vi "Build Values Tree.vi"(7 "Tree":refnum<vi>, 11 "Types":T1[](array[typedef])) -> ()   [LabVIEW 2020, in "FlexBlocks.lvlib"]
uses:
  FlexBlocks.lvlib
  Type Descriptor.ctl
  Terminal Direction.ctl
  Value Mode.ctl
  Special Terminal.ctl
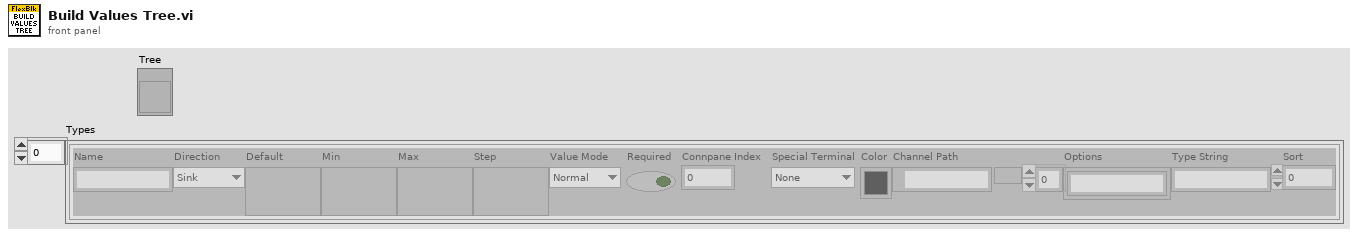
[diagram p1: front panel]
types:
  T1 = typedef "FlexBlocks.lvlib/Type Descriptor.ctl" = cluster{"Name":string, "Direction":T2, "Default":variant, "Min":variant, "Max":variant, "Step":variant, "Value Mode":T3, "Required":bool, "Connpane Index":i32, "Special Terminal":T4, "Color":u32, "Channel Path":path, "Options":string[], "Type String":string, "Sort":i32}
  T2 = typedef "FlexBlocks.lvlib/Terminal Direction.ctl" = enum16{"Sink", "Source"}
  T3 = typedef "FlexBlocks.lvlib/Value Mode.ctl" = enum16{"Normal", "Range", "Select"}
  T4 = typedef "FlexBlocks.lvlib/Special Terminal.ctl" = enum16{"None", "Action", "Init", "Tag", "State in", "State out", "Error"}
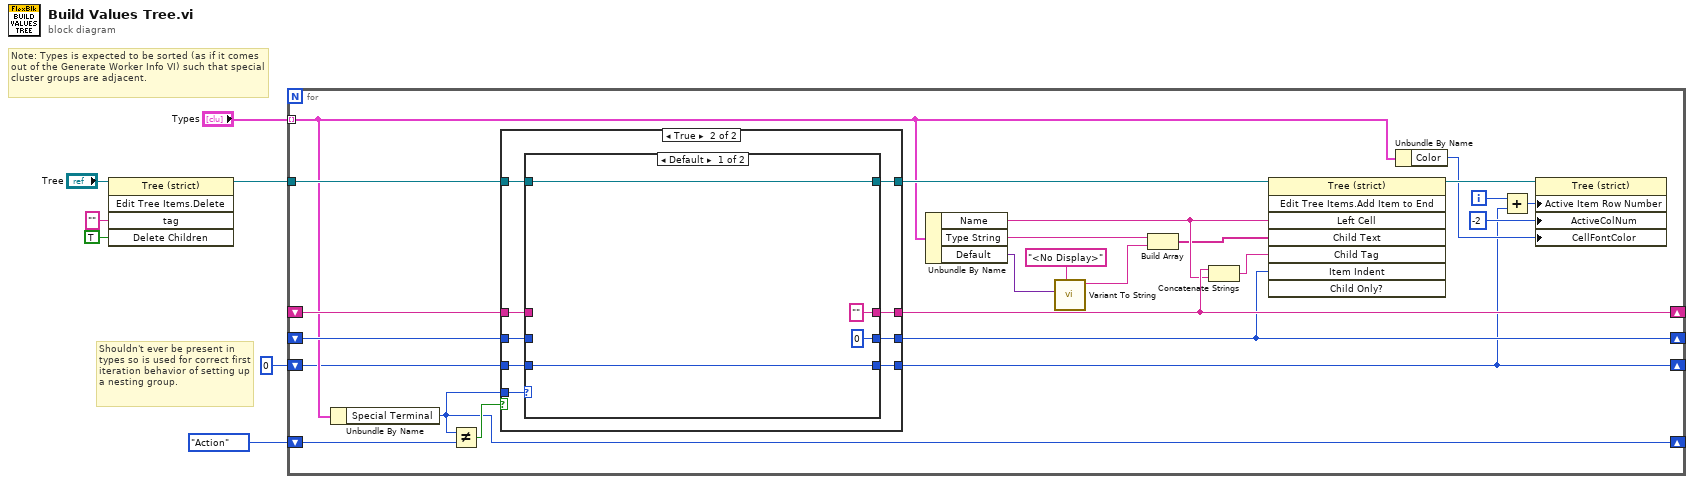
[diagram p0: block diagram]
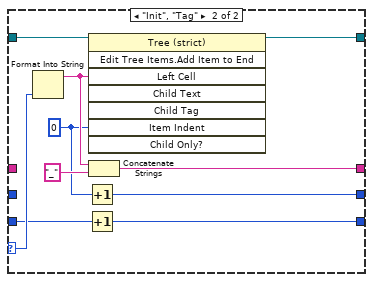
[diagram p3: hidden frame]
diagram:
  # "Shouldn't ever be present in types so is used for correct first iteration behavior of setting up a nesting group."
  # "Note: Types is expected to be sorted (as if it comes out of the Generate Worker Info VI) such that special cluster groups are adjacent."
  n1 = invoke class="Tree (strict)" method="Edit Tree Items.Delete"(reference="Tree", "tag"="" ("Tag"), "Delete Children"=TRUE ("Delete Children?")) -> (reference out=w3:refnum<vi>)  [unwired: 2 in, 4 out]
  n2 = for {
    tunnel: "Types" -> [w13] mode=indexing
    tunnel: w3 -> [w29]
    shift-right: [w28] -> _
    shift-left: Special_Terminal."Action" ("Special Terminal") -> [w31]
    shift-right: [w24] -> _
    shift-left: _ -> [w27]
    shift-right: [w21] -> _
    shift-left: _ -> [w26]
    shift-right: [w8] -> _
    shift-left: 0 -> [w11]
    i -> [w10]
    n3 = Unbundle By Name(w13) -> ("Special Terminal"=w28:T4)
    n4 = Not Equal?(x=w28, y=w31) -> (x != y?=w30:bool)
    n5 = case shown="True" w30 {
      tunnel: w29 -> [w33 w44]
      tunnel: w28 -> [_ w43]
      tunnel: [w35 w42] -> w24
      tunnel: w27 -> [w35 w41]
      tunnel: [w34 w40] -> w21
      tunnel: w26 -> [w34 w39]
      tunnel: [w33 w38] -> w25
      tunnel: w11 -> [w32 w37]
      tunnel: [w32 w36] -> w8
      frame False {
      }
      frame True {
        n6 = case shown="Default" w43 {
          selector: w43 -> [_ w57]
          tunnel: w44 -> [w46 w58]
          tunnel: ["" w54] -> w42
          tunnel: w41 -> [_ _]
          tunnel: [0 w52] -> w40
          tunnel: w39 -> [_ _]
          tunnel: [w46 w51] -> w38
          tunnel: w37 -> [w45 w50]
          tunnel: [w45 w49] -> w36
          frame Default {
          }
          frame "Init", "Tag" {
            w53 = 0 ("New Item Indentation")
            n7 = Format Into String(w57) -> (resulting string=w56:string)  [unwired: 3 in, 1 out]
            n8 = Increment(x=w53) -> (x+1=w52:i32)
            n9 = Increment(x=w50) -> (x+1=w49:i32)
            n10 = invoke class="Tree (strict)" method="Edit Tree Items.Add Item to End"(reference=w58, "Left Cell"=w56, "Item Indent"=w53) -> (reference out=w51:refnum<vi>)  [unwired: 5 in, 7 out]
            n11 = Concatenate Strings(w56, "_" ("string")) -> (w54:string)
          }
        }
      }
    }
    n12 = Unbundle By Name(w13) -> ("Name"=w23:string, "Type String"=w20:string, "Default"=w18:variant)
    n13 = call "Variant To String.vi"("Unsupported (Empty)"="<No Display>", "Variant"=w18) -> ("String"=w16:string)  [unwired: 8 in, 1 out]
    n14 = Build Array(w20, w16) -> (w19:string[])
    n15 = Concatenate Strings(w24, w23) -> (w22:string)
    n16 = invoke class="Tree (strict)" method="Edit Tree Items.Add Item to End"(reference=w25, "Left Cell"=w23, "Child Text"=w19, "Child Tag"=w22, "Item Indent"=w21) -> (reference out=w15:refnum<vi>)  [unwired: 3 in, 7 out]
    n17 = Unbundle By Name(w13) -> ("Color"=w12:u32)
    n18 = Add(x=w10, y=w8) -> (x+y=w9:i32)
    n19 = property class="Tree (strict)"(reference=w15, "Active Item Row Number"=w9, "ActiveColNum"=-2 ("Active Cell:Active Column Number"), "CellFontColor"=w12) -> ()  [unwired: 1 in, 2 out]
  }
